vi "Set Child Num.vi"(10 "Recording Cluster":T1) -> (2 "Recording Cluster out":T1)   [LabVIEW 2017, in "Digital_Group.xnode"]
uses:
  <vilib>/express/express signal manip/DigitalDataGroupingXNode/Digital_Group.xnode
  <vilib>/express/express signal manip/DigitalDataGroupingXNode/DigitalGroup_Recording Cluster.ctl
panel:
  # "This VI complete the Recording array, count the number of Lines belong to the bus"
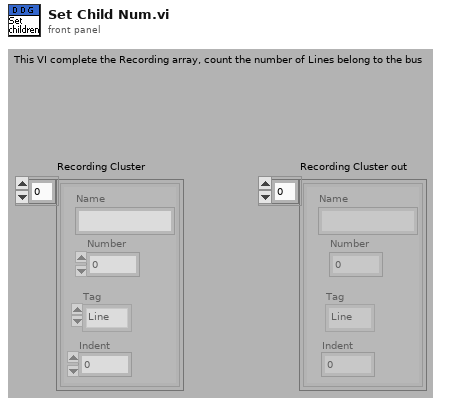
[diagram p1: front panel]
types:
  T1 = typedef "DigitalGroup_Recording Cluster.ctl" = cluster{"Name":string, "Number":u32, "Indent":u32, "Tag":enum16{"Line", "Opened Bus", "Closed Bus"}}[]
  T2 = cluster{"Name":string, "Number":u32, "Indent":u32, "Tag":enum16{"Line", "Opened Bus", "Closed Bus"}}
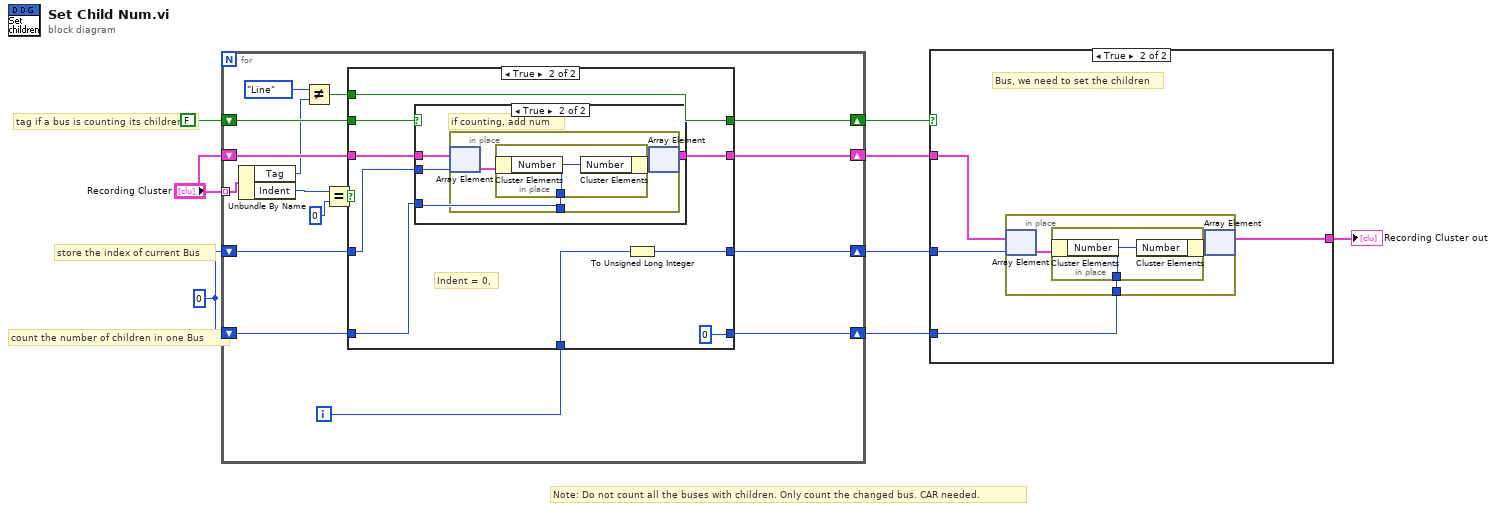
[diagram p0: block diagram]
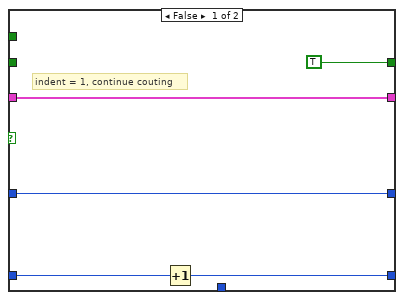
[diagram p3: hidden frame]
diagram:
  w7 = u32 0 ("Number")
  # "Note: Do not count all the buses with children. Only count the changed bus. CAR needed."
  # "tag if a bus is counting its children"
  # "store the index of current Bus"
  # "count the number of children in one Bus"
  n1 = for {
    shift-right: [w11] -> w5
    shift-left: w7 -> [w13]
    shift-right: [w23] -> w1
    shift-left: w7 -> [w22]
    shift-right: [w19] -> w6
    shift-left: "Recording Cluster" -> [w21]
    tunnel: "Recording Cluster" -> [w20] mode=indexing
    shift-right: [w9] -> w2
    shift-left: FALSE -> [w16]
    i -> [w12]
    n2 = Unbundle By Name(w20) -> ("Tag"=w15:enum16{"Line", "Opened Bus", "Closed Bus"}, "Indent"=w18:u32)
    n3 = Not Equal?(x=enum16{"Line", "Opened Bus", "Closed Bus"}."Line", y=w15) -> (x != y?=w10:bool)
    n4 = Equal?(x=w18, y=u32 0) -> (x = y?=w24:bool)
    n5 = case shown="True" w24 {
      tunnel: [w27 u32 0 ("Number")] -> w23
      tunnel: w22 -> [w28 w37]
      tunnel: w21 -> [w29 w38]
      tunnel: [w29 w36] -> w19
      tunnel: w16 -> [_ w34]
      tunnel: w13 -> [w26 w33]
      tunnel: [w26 w31] -> w11
      tunnel: w12 -> [_ w32]
      tunnel: w10 -> [_ w30]
      tunnel: [TRUE w30] -> w9
      frame False {
        # "indent = 1, continue couting"
        n6 = Increment(x=w28) -> (x+1=w27:u32)
      }
      frame True {
        # "Indent = 0,"
        n7 = case shown="True" w34 {
          tunnel: w38 -> [w39 w43]
          tunnel: w37 -> [_ w42]
          tunnel: [w39 w41] -> w36
          tunnel: w33 -> [_ w40]
          frame False {
            # "else, previous is a line, do nothing"
          }
          frame True {
            # "if counting, add num"
            n8 = in-place {
              in-place-border: w42 -> [w44]
              n9 = in-place-array #1(w43, w40) -> (w46:T2)
              n10 = in-place {
                in-place-border: w44 -> [w47]
                n11 = in-place-cluster #2(w46) -> ()  [unwired: 1 out]
                n12 = in-place-cluster #2("Number"=w47) -> (w45:T2)
              }
              n13 = in-place-array #1(w45) -> (w41:T1)  [unwired: 1 out]
            }
          }
        }
        n14 = To Unsigned Long Integer(number=w32) -> (unsigned 32bit integer=w31:u32)
      }
    }
  }
  n15 = case shown="True" w2 {
    tunnel: w6 -> [w48 w52]
    tunnel: w5 -> [_ w51]
    tunnel: [w48 w50] -> w4
    tunnel: w1 -> [_ w49]
    frame False {
    }
    frame True {
      # "Bus, we need to set the children"
      n16 = in-place {
        in-place-border: w49 -> [w53]
        n17 = in-place-array #3(w52, w51) -> (w55:T2)
        n18 = in-place {
          in-place-border: w53 -> [w56]
          n19 = in-place-cluster #4(w55) -> ()  [unwired: 1 out]
          n20 = in-place-cluster #4("Number"=w56) -> (w54:T2)
        }
        n21 = in-place-array #3(w54) -> (w50:T1)  [unwired: 1 out]
      }
    }
  }
  "Recording Cluster out" <- w4
